vi "Apply.vi"(8 "error in (no error)":errorcluster, 10 "Array in":dbl[](array[numeric]), 11 "Filter in":refnum<class "Filter.lvclass">) -> (0 "error out":errorcluster, 2 "Array out":dbl[](array[numeric]), 3 "Filter out":refnum<class "Filter.lvclass">)   [LabVIEW 2020, in "Filter.lvclass"]
uses:
  Filter.lvclass
  Filter.lvclass/Filter.ctl
  <vilib>/Analysis/3filter.llb/IIR Cascade Filter with I.C. (DBL).vi
  <vilib>/Analysis/NI_AALBase.lvlib
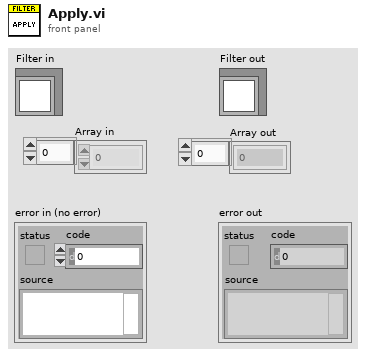
[diagram p1: front panel]
types:
  T1 = enum16{"Lowpass", "Highpass", "Bandpass", "Bandstop", "OFF"}
  T2 = typedef "Filter.lvclass/Shape.ctl" = enum16{"OFF", "Lowpass", "Highpass", "Bandpass", "Bandstop"}
  T3 = cluster{"IIR Filter":cluster{"filter structure":enum32{"IIR 2nd Order", "IIR 4th Order"}, "Reverse Coefficients":dbl[], "Forward Coefficients":dbl[]}, "State":dbl[]}[]
  T4 = cluster{"filter structure":enum32{"IIR 2nd Order", "IIR 4th Order"}, "Reverse Coefficients":dbl[], "Forward Coefficients":dbl[]}
  T5 = cluster{"IIR Filter":cluster{"filter structure":enum32{"IIR 2nd Order", "IIR 4th Order"}, "Reverse Coefficients":dbl[], "Forward Coefficients":dbl[]}, "State":dbl[]}
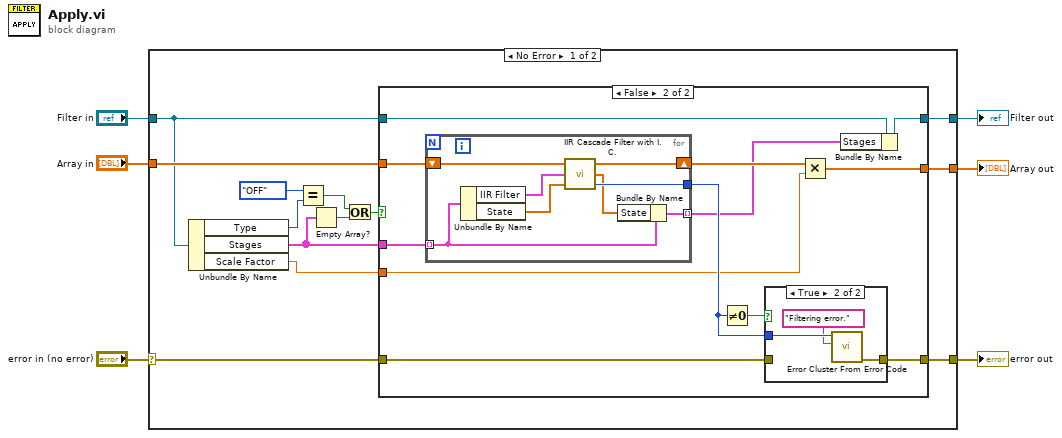
[diagram p0: block diagram]
diagram:
  n1 = case shown="No Error" "error in (no error)" {
    selector: "error in (no error)" -> [w11 w49]
    tunnel: [w10 w49] -> w5
    tunnel: [w7 w48] -> w3
    tunnel: "Filter in" -> [w8 w48]
    tunnel: [w9 w47] -> w2
    tunnel: "Array in" -> [w12 w47]
    frame No Error {
      n2 = Unbundle By Name(w8) -> ("Type"=w14:T2, "Stages"=w17:T3, "Scale Factor"=w13:dbl)
      n3 = Equal?(x=T1."OFF", y=w14) -> (x = y?=w16:bool)
      n4 = Empty Array?(array=w17) -> (empty?=w18:bool)
      n5 = Or(x=w16, y=w18) -> (x .or. y?=w19:bool)
      n6 = case shown="False" w19 {
        tunnel: w12 -> [w22 w34]
        tunnel: w17 -> [_ w23]
        tunnel: w8 -> [w20 w26]
        tunnel: [w21 w32] -> w10
        tunnel: w11 -> [w21 w30]
        tunnel: [w22 w27] -> w9
        tunnel: [w20 w24] -> w7
        tunnel: w13 -> [_ w28]
        frame True {
        }
        frame False {
          n7 = for {
            tunnel: [w41] -> w31
            shift-right: [w40] -> w29
            shift-left: w34 -> [w42]
            tunnel: w23 -> [w38] mode=indexing
            tunnel: [w36] -> w25 mode=indexing
            n8 = Unbundle By Name(w38) -> ("IIR Filter"=w39:T4, "State"=w35:dbl[])
            n9 = call-poly <vilib>:"IIR Cascade Filter with I.C..vi"("Initial Filter State"=w35, "IIR Filter Cluster"=w39, "X"=w42) -> ("error"=w41:i32, "Final Filter State"=w37:dbl[], "Filtered X"=w40:dbl[])
            n10 = Bundle By Name(cluster=w38, "State"=w37) -> (w36:T5)
          }
          n11 = Not Equal To 0?(x=w31) -> (x != 0?=w33:bool)
          n12 = case shown="True" w33 {
            tunnel: w30 -> [w43 _]
            tunnel: [w43 w45] -> w32
            tunnel: w31 -> [_ w46]
            frame False {
            }
            frame True {
              n13 = call <vilib>:"Error Cluster From Error Code.vi"("error message (\"\")"="Filtering error." ("error message (\"\")"), "error code (0)"=w46) -> ("error out"=w45:errorcluster)  [unwired: 7 in]
            }
          }
          n14 = Multiply(x=w29, y=w28) -> (x*y=w27:dbl[])
          n15 = Bundle By Name(cluster=w26, "Stages"=w25) -> (w24:refnum<class "Filter.lvclass">)
        }
      }
    }
    frame Error {
    }
  }
  "error out" <- w5
  "Filter out" <- w3
  "Array out" <- w2
